vi "Update Results.vi"(0 "measurement service in":refnum<class "IMeasurement Service.lvclass">, 5 "measurement results":variant, 7 "measurement plugin service in":refnum<class "Measurement Plugin Service.lvclass">, 9 "gRPC ID in":T1, 11 "error in":errorcluster) -> (4 "measurement service out":refnum<class "IMeasurement Service.lvclass">, 8 "measurement plugin service out":refnum<class "Measurement Plugin Service.lvclass">, 15 "error out":errorcluster)   [LabVIEW 2021, in "NI Measurement Plug-In SDK.lvlib" / "IMeasurement Service.lvclass"]
uses:
  IMeasurement Service.lvclass
  <vilib>/gRPC/LabVIEW gRPC Library/Shared/grpcId.ctl
  Measurement Plugin Service/Measurement Plugin Service.lvclass
  <vilib>/gRPC/LabVIEW gRPC Library/grpc-lvsupport-release.lvlib
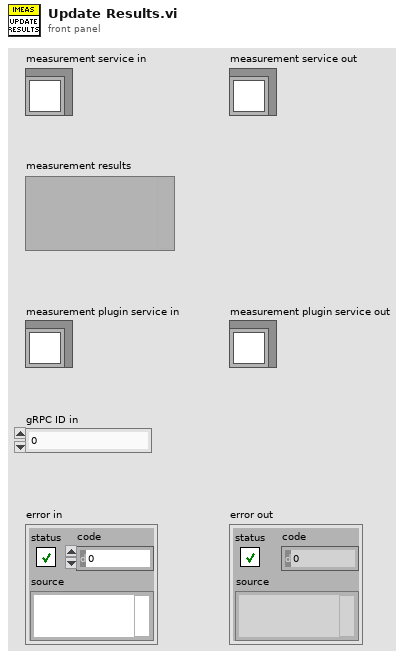
[diagram p1: front panel]
types:
  T1 = typedef "grpc-lvsupport-release.lvlib/grpcId.ctl" = u64
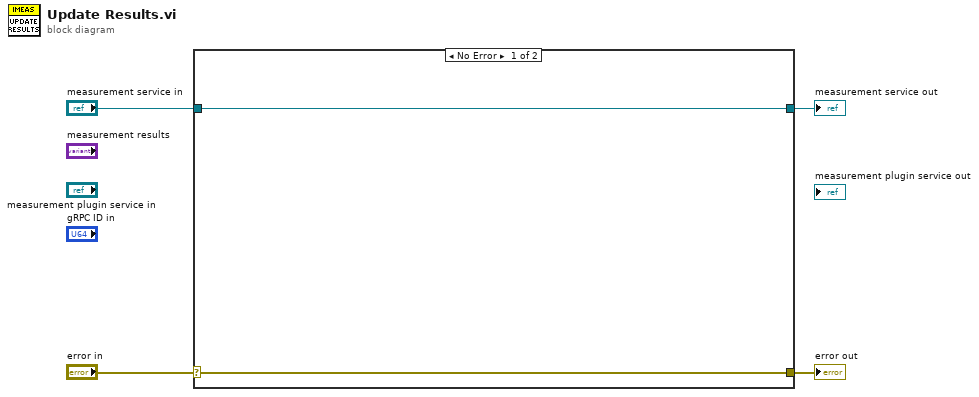
[diagram p0: block diagram]
diagram:
  n1 = case shown="No Error" "error in" {
    selector: "error in" -> [w5 w8]
    tunnel: [w5 w8] -> w3
    tunnel: [w6 w7] -> w1
    tunnel: "measurement service in" -> [w6 w7]
    frame No Error {
    }
    frame Error {
    }
  }
  "error out" <- w3
  "measurement service out" <- w1
